vi "Sensor_Save.vi"(0 "ED33_output":string[][](array[string]), 1 "Sensor_output":string[][](array[string]), 2 "ED33 Active?":bool, 3 "Current Cordinates":T1 {"Schritte B" format="%#.4g"; "Schritte A" format="%#.4g"; "Schritte C" format="%#.4g"; "Schritte U" format="%#.4g"; "Z axis" format="%#.4g"; "Y axis" format="%#.4g"; "X axis" format="%#.4g"}, 4 "Sensor Box":string(combo), 5 "Cont/MM":string(combo)="Continuous", 6 "Sensors Active?":bool, 7 "Min_move":dbl) -> ()   [LabVIEW 2013]
uses:
  <vilib>/express/express shared/transition.llb/Dynamic To Waveform Array.vi
  <vilib>/express/express signal manip/GetorSetDDTAttributes/Set DDT Attributes/SetT0.vi
  <vilib>/express/express shared/transition.llb/Waveform Array To Dynamic.vi
  <vilib>/express/express signal manip/GetorSetDDTAttributes/Set DDT Attributes/Set DDT Properties.xnode
panel:
  out "error out 2":errorcluster caption="error out"
  in  "error in (no error)":errorcluster
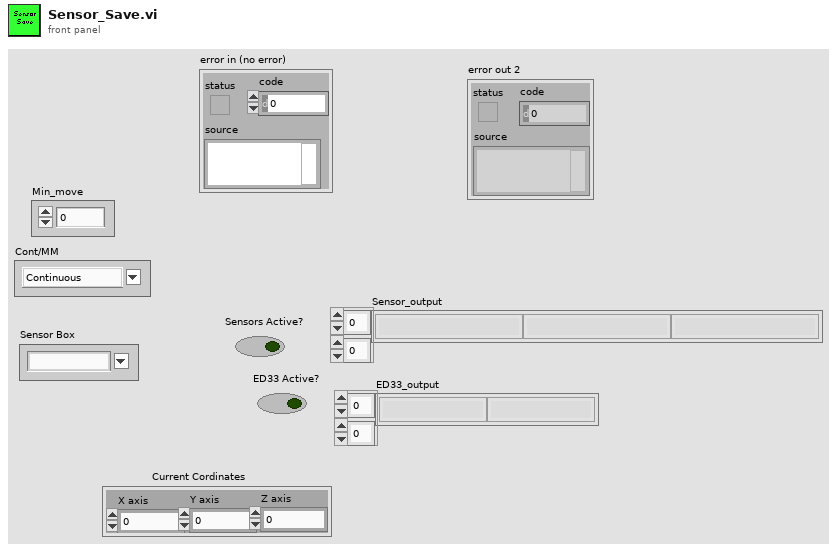
[diagram p1: front panel]
types:
  T1 = cluster{"X axis":sgl, "Y axis":sgl, "Z axis":sgl, "Schritte U":sgl, "Schritte C":sgl, "Schritte A":sgl, "Schritte B":sgl}
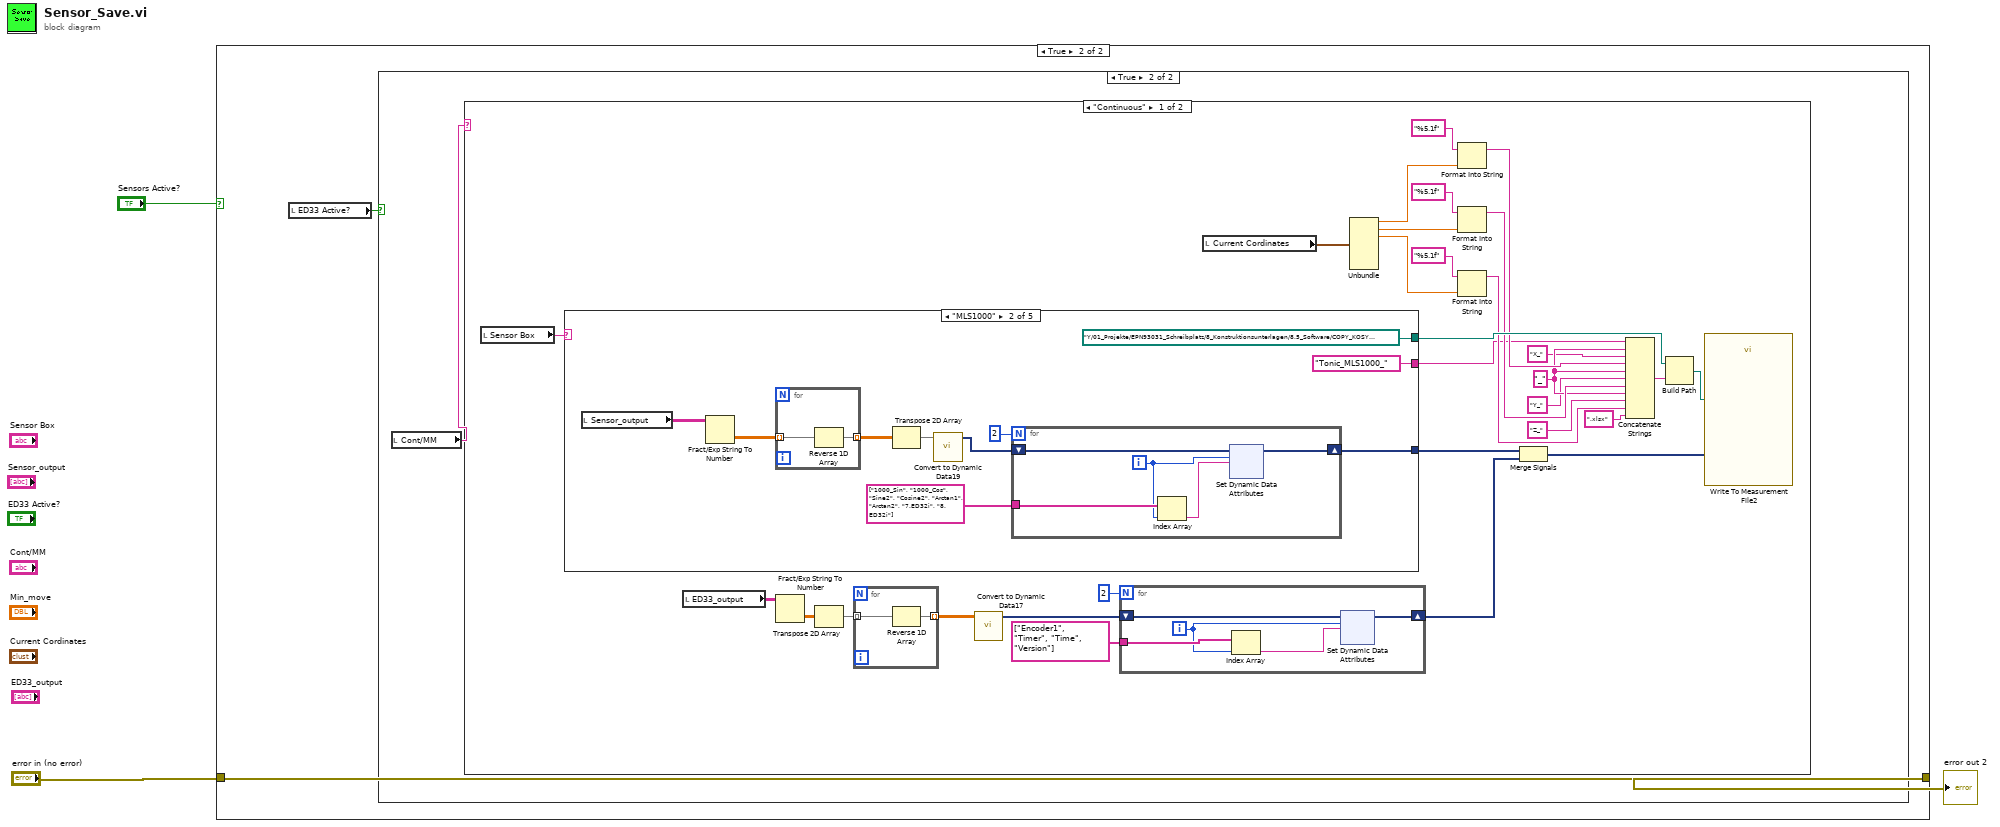
[diagram p0: block diagram]
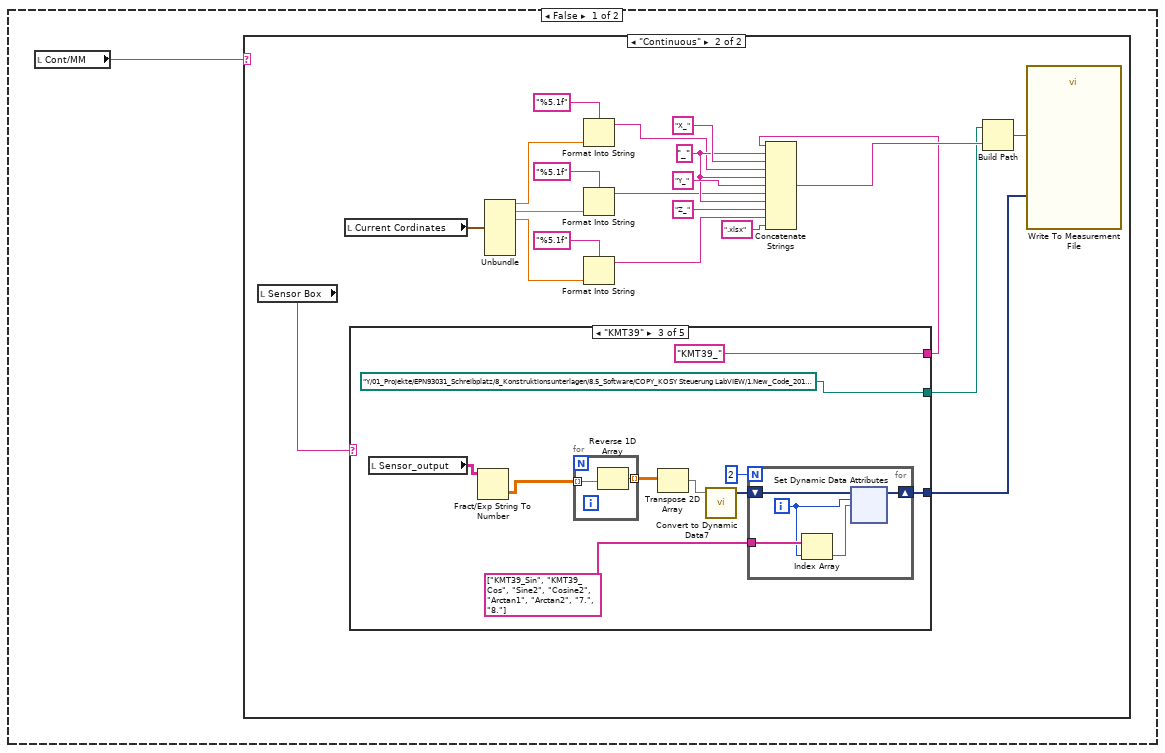
[diagram p3: hidden frame]
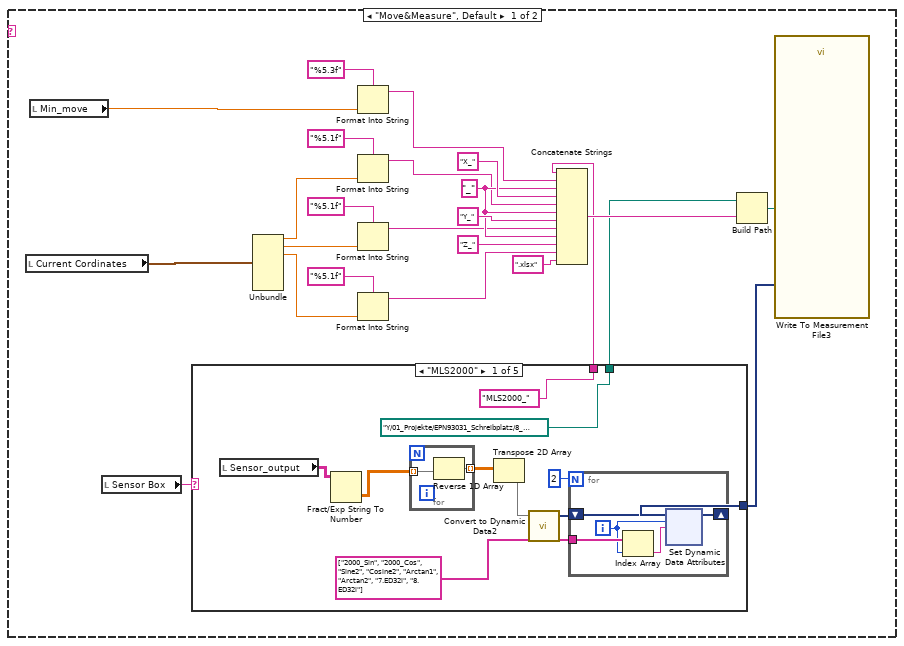
[diagram p4: hidden frame]
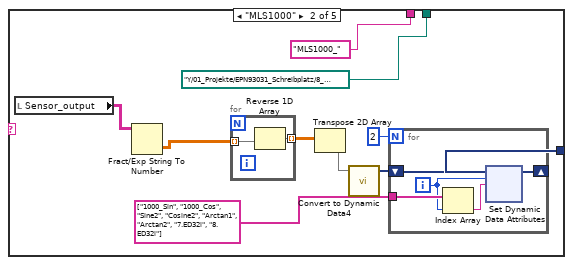
[diagram p5: hidden frame]
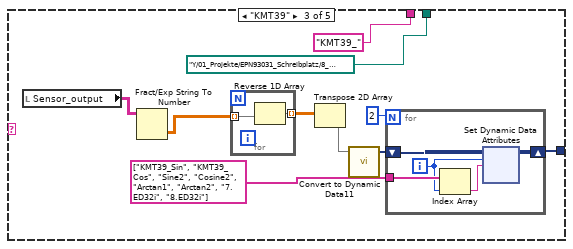
[diagram p6: hidden frame]
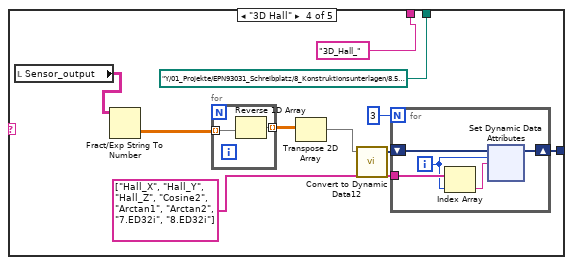
[diagram p7: hidden frame]
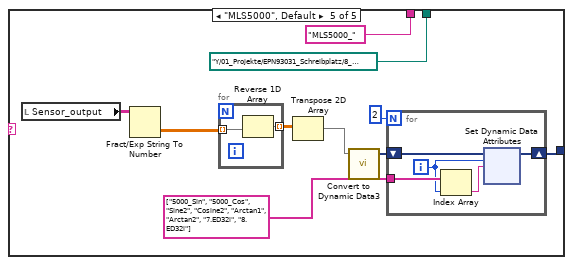
[diagram p8: hidden frame]
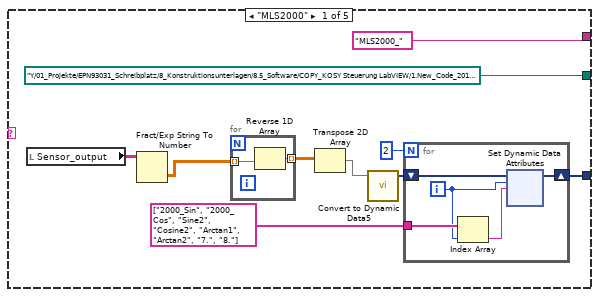
[diagram p9: hidden frame]
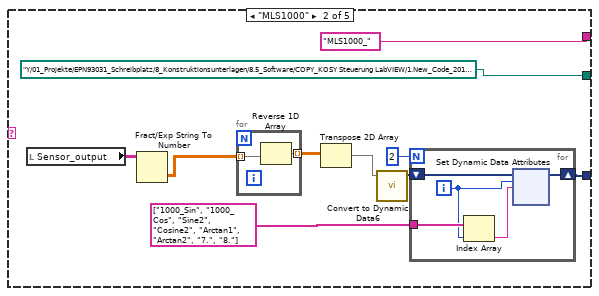
[diagram p10: hidden frame]
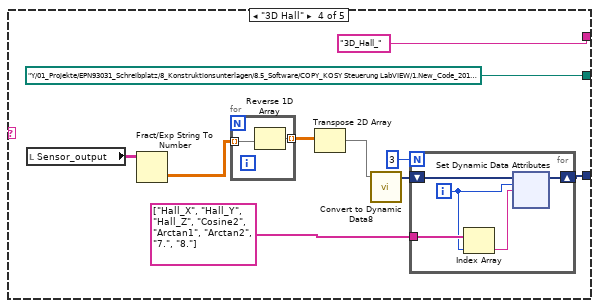
[diagram p11: hidden frame]
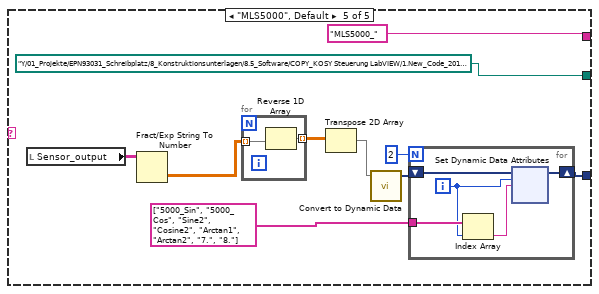
[diagram p12: hidden frame]
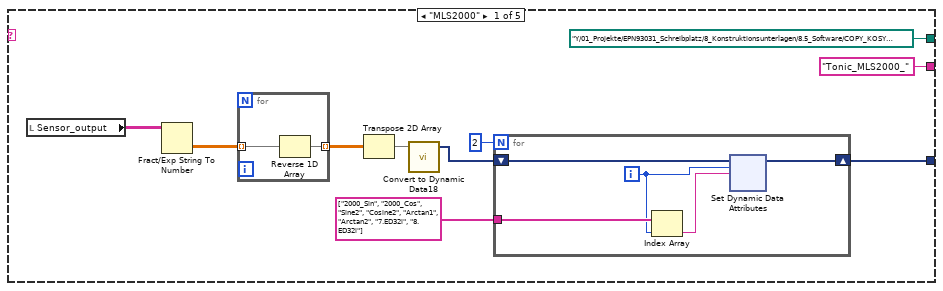
[diagram p13: hidden frame]
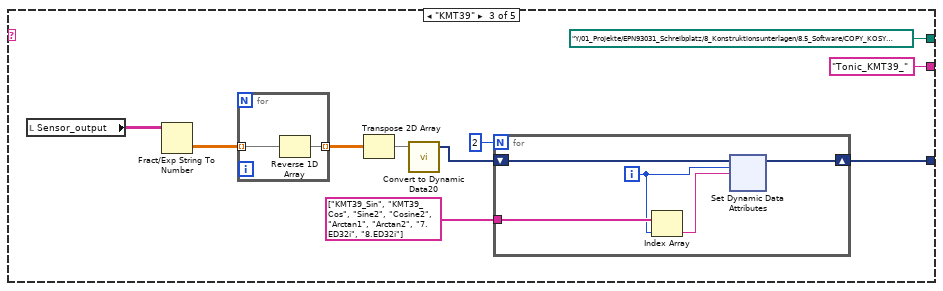
[diagram p14: hidden frame]
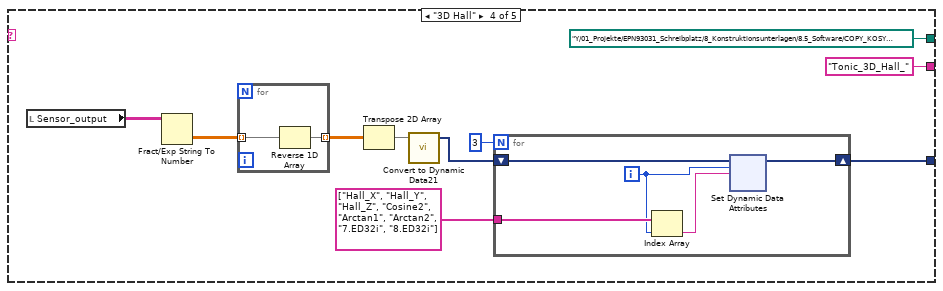
[diagram p15: hidden frame]
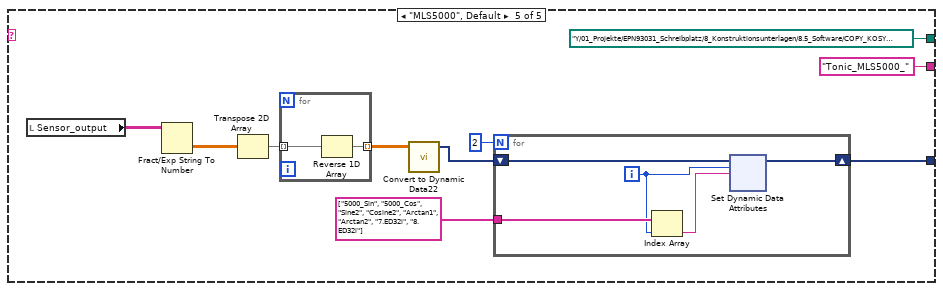
[diagram p16: hidden frame]
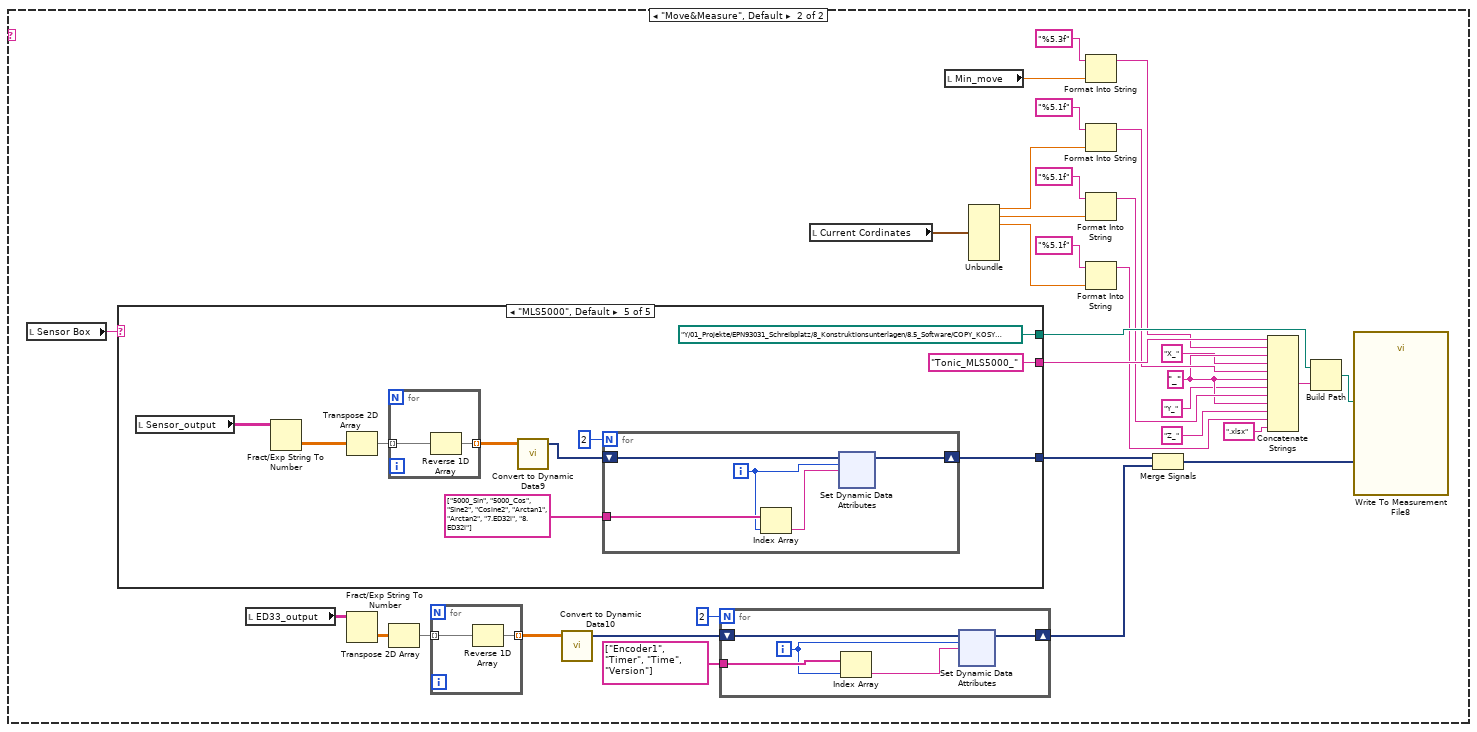
[diagram p17: hidden frame]
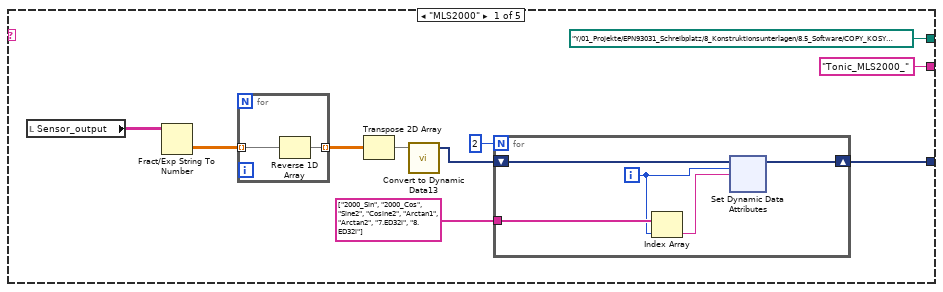
[diagram p18: hidden frame]
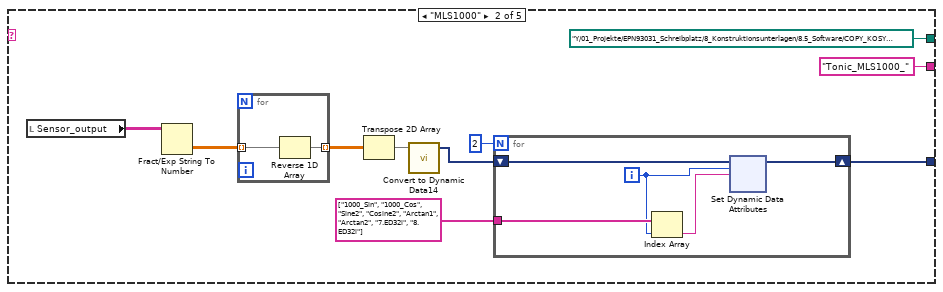
[diagram p19: hidden frame]
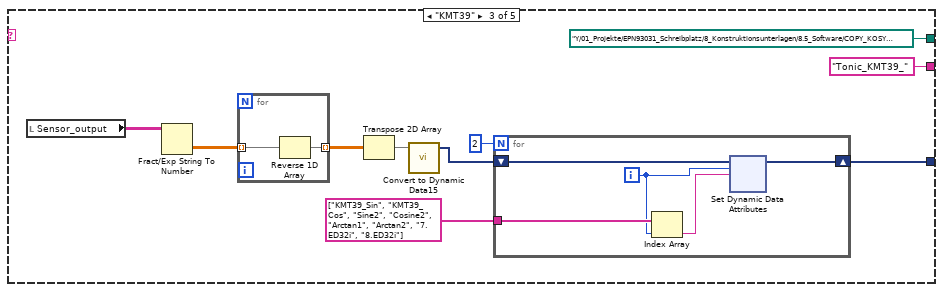
[diagram p20: hidden frame]
diagram:
  n1 = case shown="True" "Sensors Active?" {
    tunnel: "error in (no error)" -> [w4 w6]
    tunnel: [w4 w6] -> w3
    frame False {
    }
    frame True {
      n2 = local read "ED33 Active?"() -> (w5:bool)
      n3 = case shown="True" w5 {
        frame False {
          n4 = local read "Cont/MM"() -> (w7:string)
          n5 = case shown="\"Continuous\"" w7 {
            frame "Move&Measure", Default {
              w23 = "_" ("name or relative path")
              n6 = local read "Current Cordinates"() -> (w28:T1)
              n7 = local read "Min_move"() -> (w21:dbl)
              n8 = local read "Sensor Box"() -> (w10:string)
              n9 = case shown="\"MLS2000\"" w10 {
                tunnel: [w37 w67 w96 w128 w160] -> w31
                tunnel: [path "Y:/01_Projekte/EPN93031_Schreibplatz/8_Konstruktionsunterlagen/8.5_Software/COPY_KOSY Steuerung LabVIEW/1.New_Code_2014_2015/Sample_Data_ED33_32i/move&measure/MLS2000" ("base path") path "Y:/01_Projekte/EPN93031_Schreibplatz/8_Konstruktionsunterlagen/8.5_Software/COPY_KOSY Steuerung LabVIEW/1.New_Code_2014_2015/Sample_Data_ED33_32i/move&measure/MLS1000" ("base path") path "Y:/01_Projekte/EPN93031_Schreibplatz/8_Konstruktionsunterlagen/8.5_Software/COPY_KOSY Steuerung LabVIEW/1.New_Code_2014_2015/Sample_Data_ED33_32i/move&measure/KMT39" ("base path") path "Y:/01_Projekte/EPN93031_Schreibplatz/8_Konstruktionsunterlagen/8.5_Software/COPY_KOSY Steuerung LabVIEW/1.New_Code_2014_2015/Sample_Data_ED33_32i/move&measure/3D_Hall" ("base path") path "Y:/01_Projekte/EPN93031_Schreibplatz/8_Konstruktionsunterlagen/8.5_Software/COPY_KOSY Steuerung LabVIEW/1.New_Code_2014_2015/Sample_Data_ED33_32i/move&measure/MLS5000" ("base path")] -> w9
                tunnel: ["MLS2000_" ("name or relative path") "MLS1000_" ("name or relative path") "KMT39_" ("name or relative path") "3D_Hall_" ("name or relative path") "MLS5000_" ("name or relative path")] -> w8
                frame "MLS2000" {
                  n10 = local read "Sensor_output"() -> (w36:string[][])
                  n11 = Fract/Exp String To Number(string=w36) -> (number=w32:dbl[][])  [unwired: 3 in, 1 out]
                  n12 = for {
                    tunnel: w32 -> [w43] mode=indexing
                    tunnel: [w42] -> w34 mode=indexing
                    n13 = Reverse 1D Array(array=w43) -> (reversed array=w42:dbl[])
                  }
                  n14 = Transpose 2D Array(2D array=w34) -> (transposed array=w33:dbl[][])
                  n15 = call "Convert to Dynamic Data2"("2D Array"=w33) -> ("Dynamic Data Type"=w39:dynamicdata)  [unwired: 3 in]
                  n16 = for {
                    N: 2 -> [_]
                    tunnel: string[] ["2000_Sin", "2000_Cos", "Sine2", "Cosine2", "Arctan1", "Arctan2", "7.ED32i", "8.ED32i"] -> [w48]
                    shift-right: [w45] -> w37
                    shift-left: w39 -> [w44]
                    i -> [w46]
                    n17 = Index Array(array=w48, index=w46) -> (element=w47:string)
                    n18 = xnode ("Set Dynamic Data Attributes")("Signals In"=w44, "Signal Index"=w46, "Signal Name"=w47) -> ("Signals Out"=w45:dynamicdata)  [unwired: 1 in, 1 out]
                  }
                }
                frame "MLS1000" {
                  n19 = local read "Sensor_output"() -> (w68:string[][])
                  n20 = Fract/Exp String To Number(string=w68) -> (number=w62:dbl[][])  [unwired: 3 in, 1 out]
                  n21 = for {
                    tunnel: w62 -> [w73] mode=indexing
                    tunnel: [w72] -> w64 mode=indexing
                    n22 = Reverse 1D Array(array=w73) -> (reversed array=w72:dbl[])
                  }
                  n23 = Transpose 2D Array(2D array=w64) -> (transposed array=w63:dbl[][])
                  n24 = call "Convert to Dynamic Data4"("2D Array"=w63) -> ("Dynamic Data Type"=w69:dynamicdata)  [unwired: 3 in]
                  n25 = for {
                    N: 2 -> [_]
                    tunnel: string[] ["1000_Sin", "1000_Cos", "Sine2", "Cosine2", "Arctan1", "Arctan2", "7.ED32i", "8.ED32i"] -> [w78]
                    shift-right: [w75] -> w67
                    shift-left: w69 -> [w74]
                    i -> [w76]
                    n26 = Index Array(array=w78, index=w76) -> (element=w77:string)
                    n27 = xnode ("Set Dynamic Data Attributes")("Signals In"=w74, "Signal Index"=w76, "Signal Name"=w77) -> ("Signals Out"=w75:dynamicdata)  [unwired: 1 in, 1 out]
                  }
                }
                frame "KMT39" {
                  n28 = local read "Sensor_output"() -> (w98:string[][])
                  n29 = Fract/Exp String To Number(string=w98) -> (number=w92:dbl[][])  [unwired: 3 in, 1 out]
                  n30 = for {
                    tunnel: w92 -> [w103] mode=indexing
                    tunnel: [w102] -> w94 mode=indexing
                    n31 = Reverse 1D Array(array=w103) -> (reversed array=w102:dbl[])
                  }
                  n32 = Transpose 2D Array(2D array=w94) -> (transposed array=w93:dbl[][])
                  n33 = call "Convert to Dynamic Data11"("2D Array"=w93) -> ("Dynamic Data Type"=w99:dynamicdata)  [unwired: 3 in]
                  n34 = for {
                    N: 2 -> [_]
                    tunnel: string[] ["KMT39_Sin", "KMT39_Cos", "Sine2", "Cosine2", "Arctan1", "Arctan2", "7.ED32i", "8.ED32i"] -> [w108]
                    shift-right: [w105] -> w96
                    shift-left: w99 -> [w104]
                    i -> [w106]
                    n35 = Index Array(array=w108, index=w106) -> (element=w107:string)
                    n36 = xnode ("Set Dynamic Data Attributes")("Signals In"=w104, "Signal Index"=w106, "Signal Name"=w107) -> ("Signals Out"=w105:dynamicdata)  [unwired: 1 in, 1 out]
                  }
                }
                frame "3D Hall" {
                  n37 = local read "Sensor_output"() -> (w126:string[][])
                  n38 = Fract/Exp String To Number(string=w126) -> (number=w122:dbl[][])  [unwired: 3 in, 1 out]
                  n39 = for {
                    tunnel: w122 -> [w133] mode=indexing
                    tunnel: [w132] -> w124 mode=indexing
                    n40 = Reverse 1D Array(array=w133) -> (reversed array=w132:dbl[])
                  }
                  n41 = Transpose 2D Array(2D array=w124) -> (transposed array=w123:dbl[][])
                  n42 = call "Convert to Dynamic Data12"("2D Array"=w123) -> ("Dynamic Data Type"=w129:dynamicdata)  [unwired: 3 in]
                  n43 = for {
                    N: 3 -> [_]
                    tunnel: string[] ["Hall_X", "Hall_Y", "Hall_Z", "Cosine2", "Arctan1", "Arctan2", "7.ED32i", "8.ED32i"] -> [w138]
                    shift-right: [w135] -> w128
                    shift-left: w129 -> [w134]
                    i -> [w136]
                    n44 = Index Array(array=w138, index=w136) -> (element=w137:string)
                    n45 = xnode ("Set Dynamic Data Attributes")("Signals In"=w134, "Signal Index"=w136, "Signal Name"=w137) -> ("Signals Out"=w135:dynamicdata)  [unwired: 1 in, 1 out]
                  }
                }
                frame "MLS5000", Default {
                  n46 = local read "Sensor_output"() -> (w157:string[][])
                  n47 = Fract/Exp String To Number(string=w157) -> (number=w152:dbl[][])  [unwired: 3 in, 1 out]
                  n48 = for {
                    tunnel: w152 -> [w163] mode=indexing
                    tunnel: [w162] -> w154 mode=indexing
                    n49 = Reverse 1D Array(array=w163) -> (reversed array=w162:dbl[])
                  }
                  n50 = Transpose 2D Array(2D array=w154) -> (transposed array=w153:dbl[][])
                  n51 = call "Convert to Dynamic Data3"("2D Array"=w153) -> ("Dynamic Data Type"=w161:dynamicdata)  [unwired: 3 in]
                  n52 = for {
                    N: 2 -> [_]
                    tunnel: string[] ["5000_Sin", "5000_Cos", "Sine2", "Cosine2", "Arctan1", "Arctan2", "7.ED32i", "8.ED32i"] -> [w168]
                    shift-right: [w165] -> w160
                    shift-left: w161 -> [w164]
                    i -> [w166]
                    n53 = Index Array(array=w168, index=w166) -> (element=w167:string)
                    n54 = xnode ("Set Dynamic Data Attributes")("Signals In"=w164, "Signal Index"=w166, "Signal Name"=w167) -> ("Signals Out"=w165:dynamicdata)  [unwired: 1 in, 1 out]
                  }
                }
              }
              n55 = Unbundle(w28) -> ("X axis"=w16:sgl, "Y axis"=w15:sgl, "Z axis"=w14:sgl)  [unwired: 4 out]
              n56 = Format Into String(format string="%5.3f", w21) -> (resulting string=w20:string)  [unwired: 2 in, 1 out]
              n57 = Format Into String(format string="%5.1f", w16) -> (resulting string=w13:string)  [unwired: 2 in, 1 out]
              n58 = Format Into String(format string="%5.1f", w15) -> (resulting string=w12:string)  [unwired: 2 in, 1 out]
              n59 = Format Into String(format string="%5.1f", w14) -> (resulting string=w11:string)  [unwired: 2 in, 1 out]
              n60 = Concatenate Strings(w8, w20, w23, "X_" ("name or relative path"), w13, w23, "Y_" ("name or relative path"), w12, w23, "Z_" ("name or relative path"), w11, ".xlsx" ("name or relative path")) -> (w30:string)
              n61 = Build Path(base path=w9, name or relative path=w30) -> (appended path=w29:path)
              n62 = call "Write To Measurement File3"("Signals"=w31, "Filename"=w29) -> ()  [unwired: 15 in, 3 out]
            }
            frame "Continuous" {
              w196 = "_" ("name or relative path")
              n63 = local read "Sensor Box"() -> (w184:string)
              n64 = local read "Current Cordinates"() -> (w186:T1)
              n65 = case shown="\"KMT39\"" w184 {
                tunnel: [w208 w238 w269 w298 w331] -> w202
                tunnel: [path "Y:/01_Projekte/EPN93031_Schreibplatz/8_Konstruktionsunterlagen/8.5_Software/COPY_KOSY Steuerung LabVIEW/1.New_Code_2014_2015/Sample_Data_ED33_32i/continuous/MLS2000" ("base path") path "Y:/01_Projekte/EPN93031_Schreibplatz/8_Konstruktionsunterlagen/8.5_Software/COPY_KOSY Steuerung LabVIEW/1.New_Code_2014_2015/Sample_Data_ED33_32i/continuous/MLS1000" ("base path") path "Y:/01_Projekte/EPN93031_Schreibplatz/8_Konstruktionsunterlagen/8.5_Software/COPY_KOSY Steuerung LabVIEW/1.New_Code_2014_2015/Sample_Data_ED33_32i/continuous/KMT39" ("base path") path "Y:/01_Projekte/EPN93031_Schreibplatz/8_Konstruktionsunterlagen/8.5_Software/COPY_KOSY Steuerung LabVIEW/1.New_Code_2014_2015/Sample_Data_ED33_32i/continuous/3D_Hall" ("base path") path "Y:/01_Projekte/EPN93031_Schreibplatz/8_Konstruktionsunterlagen/8.5_Software/COPY_KOSY Steuerung LabVIEW/1.New_Code_2014_2015/Sample_Data_ED33_32i/continuous/MLS5000" ("base path")] -> w183
                tunnel: ["MLS2000_" ("name or relative path") "MLS1000_" ("name or relative path") "KMT39_" ("name or relative path") "3D_Hall_" ("name or relative path") "MLS5000_" ("name or relative path")] -> w182
                frame "MLS2000" {
                  n66 = local read "Sensor_output"() -> (w209:string[][])
                  n67 = Fract/Exp String To Number(string=w209) -> (number=w203:dbl[][])  [unwired: 3 in, 1 out]
                  n68 = for {
                    tunnel: w203 -> [w214] mode=indexing
                    tunnel: [w213] -> w205 mode=indexing
                    n69 = Reverse 1D Array(array=w214) -> (reversed array=w213:dbl[])
                  }
                  n70 = Transpose 2D Array(2D array=w205) -> (transposed array=w204:dbl[][])
                  n71 = call "Convert to Dynamic Data5"("2D Array"=w204) -> ("Dynamic Data Type"=w212:dynamicdata)  [unwired: 3 in]
                  n72 = for {
                    N: 2 -> [_]
                    tunnel: string[] ["2000_Sin", "2000_Cos", "Sine2", "Cosine2", "Arctan1", "Arctan2", "7.", "8."] -> [w219]
                    shift-right: [w216] -> w208
                    shift-left: w212 -> [w215]
                    i -> [w217]
                    n73 = Index Array(array=w219, index=w217) -> (element=w218:string)
                    n74 = xnode ("Set Dynamic Data Attributes")("Signals In"=w215, "Signal Index"=w217, "Signal Name"=w218) -> ("Signals Out"=w216:dynamicdata)  [unwired: 1 in, 1 out]
                  }
                }
                frame "MLS1000" {
                  n75 = local read "Sensor_output"() -> (w239:string[][])
                  n76 = Fract/Exp String To Number(string=w239) -> (number=w233:dbl[][])  [unwired: 3 in, 1 out]
                  n77 = for {
                    tunnel: w233 -> [w244] mode=indexing
                    tunnel: [w243] -> w235 mode=indexing
                    n78 = Reverse 1D Array(array=w244) -> (reversed array=w243:dbl[])
                  }
                  n79 = Transpose 2D Array(2D array=w235) -> (transposed array=w234:dbl[][])
                  n80 = call "Convert to Dynamic Data6"("2D Array"=w234) -> ("Dynamic Data Type"=w242:dynamicdata)  [unwired: 3 in]
                  n81 = for {
                    N: 2 -> [_]
                    tunnel: string[] ["1000_Sin", "1000_Cos", "Sine2", "Cosine2", "Arctan1", "Arctan2", "7.", "8."] -> [w249]
                    shift-right: [w246] -> w238
                    shift-left: w242 -> [w245]
                    i -> [w247]
                    n82 = Index Array(array=w249, index=w247) -> (element=w248:string)
                    n83 = xnode ("Set Dynamic Data Attributes")("Signals In"=w245, "Signal Index"=w247, "Signal Name"=w248) -> ("Signals Out"=w246:dynamicdata)  [unwired: 1 in, 1 out]
                  }
                }
                frame "KMT39" {
                  n84 = local read "Sensor_output"() -> (w266:string[][])
                  n85 = Fract/Exp String To Number(string=w266) -> (number=w263:dbl[][])  [unwired: 3 in, 1 out]
                  n86 = for {
                    tunnel: w263 -> [w274] mode=indexing
                    tunnel: [w273] -> w265 mode=indexing
                    n87 = Reverse 1D Array(array=w274) -> (reversed array=w273:dbl[])
                  }
                  n88 = Transpose 2D Array(2D array=w265) -> (transposed array=w264:dbl[][])
                  n89 = call "Convert to Dynamic Data7"("2D Array"=w264) -> ("Dynamic Data Type"=w270:dynamicdata)  [unwired: 3 in]
                  n90 = for {
                    N: 2 -> [_]
                    tunnel: string[] ["KMT39_Sin", "KMT39_Cos", "Sine2", "Cosine2", "Arctan1", "Arctan2", "7.", "8."] -> [w279]
                    shift-right: [w276] -> w269
                    shift-left: w270 -> [w275]
                    i -> [w277]
                    n91 = Index Array(array=w279, index=w277) -> (element=w278:string)
                    n92 = xnode ("Set Dynamic Data Attributes")("Signals In"=w275, "Signal Index"=w277, "Signal Name"=w278) -> ("Signals Out"=w276:dynamicdata)  [unwired: 1 in, 1 out]
                  }
                }
                frame "3D Hall" {
                  n93 = local read "Sensor_output"() -> (w299:string[][])
                  n94 = Fract/Exp String To Number(string=w299) -> (number=w293:dbl[][])  [unwired: 3 in, 1 out]
                  n95 = for {
                    tunnel: w293 -> [w304] mode=indexing
                    tunnel: [w303] -> w295 mode=indexing
                    n96 = Reverse 1D Array(array=w304) -> (reversed array=w303:dbl[])
                  }
                  n97 = Transpose 2D Array(2D array=w295) -> (transposed array=w294:dbl[][])
                  n98 = call "Convert to Dynamic Data8"("2D Array"=w294) -> ("Dynamic Data Type"=w302:dynamicdata)  [unwired: 3 in]
                  n99 = for {
                    N: 3 -> [_]
                    tunnel: string[] ["Hall_X", "Hall_Y", "Hall_Z", "Cosine2", "Arctan1", "Arctan2", "7.", "8."] -> [w309]
                    shift-right: [w306] -> w298
                    shift-left: w302 -> [w305]
                    i -> [w307]
                    n100 = Index Array(array=w309, index=w307) -> (element=w308:string)
                    n101 = xnode ("Set Dynamic Data Attributes")("Signals In"=w305, "Signal Index"=w307, "Signal Name"=w308) -> ("Signals Out"=w306:dynamicdata)  [unwired: 1 in, 1 out]
                  }
                }
                frame "MLS5000", Default {
                  n102 = local read "Sensor_output"() -> (w328:string[][])
                  n103 = Fract/Exp String To Number(string=w328) -> (number=w323:dbl[][])  [unwired: 3 in, 1 out]
                  n104 = for {
                    tunnel: w323 -> [w334] mode=indexing
                    tunnel: [w333] -> w325 mode=indexing
                    n105 = Reverse 1D Array(array=w334) -> (reversed array=w333:dbl[])
                  }
                  n106 = Transpose 2D Array(2D array=w325) -> (transposed array=w324:dbl[][])
                  n107 = call "Convert to Dynamic Data"("2D Array"=w324) -> ("Dynamic Data Type"=w332:dynamicdata)  [unwired: 3 in]
                  n108 = for {
                    N: 2 -> [_]
                    tunnel: string[] ["5000_Sin", "5000_Cos", "Sine2", "Cosine2", "Arctan1", "Arctan2", "7.", "8."] -> [w339]
                    shift-right: [w336] -> w331
                    shift-left: w332 -> [w335]
                    i -> [w337]
                    n109 = Index Array(array=w339, index=w337) -> (element=w338:string)
                    n110 = xnode ("Set Dynamic Data Attributes")("Signals In"=w335, "Signal Index"=w337, "Signal Name"=w338) -> ("Signals Out"=w336:dynamicdata)  [unwired: 1 in, 1 out]
                  }
                }
              }
              n111 = Unbundle(w186) -> ("X axis"=w192:sgl, "Y axis"=w191:sgl, "Z axis"=w190:sgl)  [unwired: 4 out]
              n112 = Format Into String(format string="%5.1f", w192) -> (resulting string=w189:string)  [unwired: 2 in, 1 out]
              n113 = Format Into String(format string="%5.1f", w191) -> (resulting string=w188:string)  [unwired: 2 in, 1 out]
              n114 = Format Into String(format string="%5.1f", w190) -> (resulting string=w187:string)  [unwired: 2 in, 1 out]
              n115 = Concatenate Strings(w182, w196, "X_" ("name or relative path"), w189, w196, "Y_" ("name or relative path"), w188, w196, "Z_" ("name or relative path"), w187, ".xlsx" ("name or relative path")) -> (w201:string)
              n116 = Build Path(base path=w183, name or relative path=w201) -> (appended path=w185:path)
              n117 = call "Write To Measurement File"("Signals"=w202, "Filename"=w185) -> ()  [unwired: 15 in, 3 out]
            }
          }
        }
        frame True {
          n118 = local read "Cont/MM"() -> (w353:string)
          n119 = case shown="\"Continuous\"" w353 {
            frame "Continuous" {
              w371 = "_" ("name or relative path")
              n120 = local read "Sensor Box"() -> (w365:string)
              n121 = case shown="\"MLS1000\"" w365 {
                tunnel: [w392 w421 w451 w481 w515] -> w359
                tunnel: [path "Y:/01_Projekte/EPN93031_Schreibplatz/8_Konstruktionsunterlagen/8.5_Software/COPY_KOSY Steuerung LabVIEW/1.New_Code_2014_2015/Sample_Data_ED33_32i/continuous/With_Ref/MLS2000" ("base path") path "Y:/01_Projekte/EPN93031_Schreibplatz/8_Konstruktionsunterlagen/8.5_Software/COPY_KOSY Steuerung LabVIEW/1.New_Code_2014_2015/Sample_Data_ED33_32i/continuous/With_Ref/MLS1000" ("base path") path "Y:/01_Projekte/EPN93031_Schreibplatz/8_Konstruktionsunterlagen/8.5_Software/COPY_KOSY Steuerung LabVIEW/1.New_Code_2014_2015/Sample_Data_ED33_32i/continuous/With_Ref/KMT39" ("base path") path "Y:/01_Projekte/EPN93031_Schreibplatz/8_Konstruktionsunterlagen/8.5_Software/COPY_KOSY Steuerung LabVIEW/1.New_Code_2014_2015/Sample_Data_ED33_32i/continuous/With_Ref/3D_Hall" ("base path") path "Y:/01_Projekte/EPN93031_Schreibplatz/8_Konstruktionsunterlagen/8.5_Software/COPY_KOSY Steuerung LabVIEW/1.New_Code_2014_2015/Sample_Data_ED33_32i/continuous/With_Ref/MLS5000" ("base path")] -> w382
                tunnel: ["Tonic_MLS2000_" ("name or relative path") "Tonic_MLS1000_" ("name or relative path") "Tonic_KMT39_" ("name or relative path") "Tonic_3D_Hall_" ("name or relative path") "Tonic_MLS5000_" ("name or relative path")] -> w354
                frame "MLS2000" {
                  n122 = local read "Sensor_output"() -> (w391:string[][])
                  n123 = Fract/Exp String To Number(string=w391) -> (number=w386:dbl[][])  [unwired: 3 in, 1 out]
                  n124 = for {
                    tunnel: w386 -> [w397] mode=indexing
                    tunnel: [w396] -> w388 mode=indexing
                    n125 = Reverse 1D Array(array=w397) -> (reversed array=w396:dbl[])
                  }
                  n126 = Transpose 2D Array(2D array=w388) -> (transposed array=w387:dbl[][])
                  n127 = call "Convert to Dynamic Data18"("2D Array"=w387) -> ("Dynamic Data Type"=w394:dynamicdata)  [unwired: 3 in]
                  n128 = for {
                    N: 2 -> [_]
                    tunnel: string[] ["2000_Sin", "2000_Cos", "Sine2", "Cosine2", "Arctan1", "Arctan2", "7.ED32i", "8.ED32i"] -> [w402]
                    shift-right: [w399] -> w392
                    shift-left: w394 -> [w398]
                    i -> [w400]
                    n129 = Index Array(array=w402, index=w400) -> (element=w401:string)
                    n130 = xnode ("Set Dynamic Data Attributes")("Signals In"=w398, "Signal Index"=w400, "Signal Name"=w401) -> ("Signals Out"=w399:dynamicdata)  [unwired: 1 in, 1 out]
                  }
                }
                frame "MLS1000" {
                  n131 = local read "Sensor_output"() -> (w422:string[][])
                  n132 = Fract/Exp String To Number(string=w422) -> (number=w416:dbl[][])  [unwired: 3 in, 1 out]
                  n133 = for {
                    tunnel: w416 -> [w427] mode=indexing
                    tunnel: [w426] -> w418 mode=indexing
                    n134 = Reverse 1D Array(array=w427) -> (reversed array=w426:dbl[])
                  }
                  n135 = Transpose 2D Array(2D array=w418) -> (transposed array=w417:dbl[][])
                  n136 = call "Convert to Dynamic Data19"("2D Array"=w417) -> ("Dynamic Data Type"=w424:dynamicdata)  [unwired: 3 in]
                  n137 = for {
                    N: 2 -> [_]
                    tunnel: string[] ["1000_Sin", "1000_Cos", "Sine2", "Cosine2", "Arctan1", "Arctan2", "7.ED32i", "8.ED32i"] -> [w432]
                    shift-right: [w429] -> w421
                    shift-left: w424 -> [w428]
                    i -> [w430]
                    n138 = Index Array(array=w432, index=w430) -> (element=w431:string)
                    n139 = xnode ("Set Dynamic Data Attributes")("Signals In"=w428, "Signal Index"=w430, "Signal Name"=w431) -> ("Signals Out"=w429:dynamicdata)  [unwired: 1 in, 1 out]
                  }
                }
                frame "KMT39" {
                  n140 = local read "Sensor_output"() -> (w452:string[][])
                  n141 = Fract/Exp String To Number(string=w452) -> (number=w446:dbl[][])  [unwired: 3 in, 1 out]
                  n142 = for {
                    tunnel: w446 -> [w457] mode=indexing
                    tunnel: [w456] -> w448 mode=indexing
                    n143 = Reverse 1D Array(array=w457) -> (reversed array=w456:dbl[])
                  }
                  n144 = Transpose 2D Array(2D array=w448) -> (transposed array=w447:dbl[][])
                  n145 = call "Convert to Dynamic Data20"("2D Array"=w447) -> ("Dynamic Data Type"=w454:dynamicdata)  [unwired: 3 in]
                  n146 = for {
                    N: 2 -> [_]
                    tunnel: string[] ["KMT39_Sin", "KMT39_Cos", "Sine2", "Cosine2", "Arctan1", "Arctan2", "7.ED32i", "8.ED32i"] -> [w462]
                    shift-right: [w459] -> w451
                    shift-left: w454 -> [w458]
                    i -> [w460]
                    n147 = Index Array(array=w462, index=w460) -> (element=w461:string)
                    n148 = xnode ("Set Dynamic Data Attributes")("Signals In"=w458, "Signal Index"=w460, "Signal Name"=w461) -> ("Signals Out"=w459:dynamicdata)  [unwired: 1 in, 1 out]
                  }
                }
                frame "3D Hall" {
                  n149 = local read "Sensor_output"() -> (w482:string[][])
                  n150 = Fract/Exp String To Number(string=w482) -> (number=w476:dbl[][])  [unwired: 3 in, 1 out]
                  n151 = for {
                    tunnel: w476 -> [w487] mode=indexing
                    tunnel: [w486] -> w478 mode=indexing
                    n152 = Reverse 1D Array(array=w487) -> (reversed array=w486:dbl[])
                  }
                  n153 = Transpose 2D Array(2D array=w478) -> (transposed array=w477:dbl[][])
                  n154 = call "Convert to Dynamic Data21"("2D Array"=w477) -> ("Dynamic Data Type"=w484:dynamicdata)  [unwired: 3 in]
                  n155 = for {
                    N: 3 -> [_]
                    tunnel: string[] ["Hall_X", "Hall_Y", "Hall_Z", "Cosine2", "Arctan1", "Arctan2", "7.ED32i", "8.ED32i"] -> [w492]
                    shift-right: [w489] -> w481
                    shift-left: w484 -> [w488]
                    i -> [w490]
                    n156 = Index Array(array=w492, index=w490) -> (element=w491:string)
                    n157 = xnode ("Set Dynamic Data Attributes")("Signals In"=w488, "Signal Index"=w490, "Signal Name"=w491) -> ("Signals Out"=w489:dynamicdata)  [unwired: 1 in, 1 out]
                  }
                }
                frame "MLS5000", Default {
                  n158 = local read "Sensor_output"() -> (w514:string[][])
                  n159 = Fract/Exp String To Number(string=w514) -> (number=w507:dbl[][])  [unwired: 3 in, 1 out]
                  n160 = Transpose 2D Array(2D array=w507) -> (transposed array=w506:dbl[][])
                  n161 = for {
                    tunnel: w506 -> [w517] mode=indexing
                    tunnel: [w516] -> w508 mode=indexing
                    n162 = Reverse 1D Array(array=w517) -> (reversed array=w516:dbl[])
                  }
                  n163 = call "Convert to Dynamic Data22"("2D Array"=w508) -> ("Dynamic Data Type"=w512:dynamicdata)  [unwired: 3 in]
                  n164 = for {
                    N: 2 -> [_]
                    tunnel: string[] ["5000_Sin", "5000_Cos", "Sine2", "Cosine2", "Arctan1", "Arctan2", "7.ED32i", "8.ED32i"] -> [w522]
                    shift-right: [w519] -> w515
                    shift-left: w512 -> [w518]
                    i -> [w520]
                    n165 = Index Array(array=w522, index=w520) -> (element=w521:string)
                    n166 = xnode ("Set Dynamic Data Attributes")("Signals In"=w518, "Signal Index"=w520, "Signal Name"=w521) -> ("Signals Out"=w519:dynamicdata)  [unwired: 1 in, 1 out]
                  }
                }
              }
              n167 = local read "ED33_output"() -> (w361:string[][])
              n168 = Fract/Exp String To Number(string=w361) -> (number=w356:dbl[][])  [unwired: 3 in, 1 out]
              n169 = Transpose 2D Array(2D array=w356) -> (transposed array=w355:dbl[][])
              n170 = for {
                tunnel: w355 -> [w385] mode=indexing
                tunnel: [w384] -> w357 mode=indexing
                n171 = Reverse 1D Array(array=w385) -> (reversed array=w384:dbl[])
              }
              n172 = call "Convert to Dynamic Data17"("2D Array"=w357) -> ("Dynamic Data Type"=w362:dynamicdata)  [unwired: 3 in]
              n173 = for {
                N: 2 -> [_]
                tunnel: string[] ["Encoder1", "Timer", "Time", "Version"] -> [w540]
                shift-right: [w537] -> w360
                shift-left: w362 -> [w536]
                i -> [w538]
                n174 = Index Array(array=w540, index=w538) -> (element=w539:string)
                n175 = xnode ("Set Dynamic Data Attributes")("Signals In"=w536, "Signal Index"=w538, "Signal Name"=w539) -> ("Signals Out"=w537:dynamicdata)  [unwired: 1 in, 1 out]
              }
              n176 = local read "Current Cordinates"() -> (w381:T1)
              n177 = Unbundle(w381) -> ("X axis"=w375:sgl, "Y axis"=w376:sgl, "Z axis"=w377:sgl)  [unwired: 4 out]
              n178 = Format Into String(format string="%5.1f", w375) -> (resulting string=w378:string)  [unwired: 2 in, 1 out]
              n179 = Format Into String(format string="%5.1f", w376) -> (resulting string=w379:string)  [unwired: 2 in, 1 out]
              n180 = Format Into String(format string="%5.1f", w377) -> (resulting string=w380:string)  [unwired: 2 in, 1 out]
              n181 = Merge Signals(w359, w360) -> (w358:dynamicdata)
              n182 = Concatenate Strings(w354, w371, "X_" ("name or relative path"), w378, w371, "Y_" ("name or relative path"), w379, w371, "Z_" ("name or relative path"), w380, ".xlsx" ("name or relative path")) -> (w366:string)
              n183 = Build Path(base path=w382, name or relative path=w366) -> (appended path=w383:path)
              n184 = call "Write To Measurement File2"("Signals"=w358, "Filename"=w383) -> ()  [unwired: 15 in, 3 out]
            }
            frame "Move&Measure", Default {
              w570 = "_" ("name or relative path")
              n185 = local read "Sensor Box"() -> (w564:string)
              n186 = case shown="\"MLS5000\", Default" w564 {
                tunnel: [w595 w624 w654 w684 w718] -> w558
                tunnel: [path "Y:/01_Projekte/EPN93031_Schreibplatz/8_Konstruktionsunterlagen/8.5_Software/COPY_KOSY Steuerung LabVIEW/1.New_Code_2014_2015/Sample_Data_ED33_32i/move&measure/With_Ref/MLS2000" ("base path") path "Y:/01_Projekte/EPN93031_Schreibplatz/8_Konstruktionsunterlagen/8.5_Software/COPY_KOSY Steuerung LabVIEW/1.New_Code_2014_2015/Sample_Data_ED33_32i/move&measure/With_Ref/MLS1000" ("base path") path "Y:/01_Projekte/EPN93031_Schreibplatz/8_Konstruktionsunterlagen/8.5_Software/COPY_KOSY Steuerung LabVIEW/1.New_Code_2014_2015/Sample_Data_ED33_32i/move&measure/With_Ref/KMT39" ("base path") path "Y:/01_Projekte/EPN93031_Schreibplatz/8_Konstruktionsunterlagen/8.5_Software/COPY_KOSY Steuerung LabVIEW/1.New_Code_2014_2015/Sample_Data_ED33_32i/move&measure/With_Ref/3D_Hall" ("base path") path "Y:/01_Projekte/EPN93031_Schreibplatz/8_Konstruktionsunterlagen/8.5_Software/COPY_KOSY Steuerung LabVIEW/1.New_Code_2014_2015/Sample_Data_ED33_32i/move&measure/With_Ref/MLS5000" ("base path")] -> w584
                tunnel: ["Tonic_MLS2000_" ("name or relative path") "Tonic_MLS1000_" ("name or relative path") "Tonic_KMT39_" ("name or relative path") "Tonic_3D_Hall_" ("name or relative path") "Tonic_MLS5000_" ("name or relative path")] -> w585
                frame "MLS2000" {
                  n187 = local read "Sensor_output"() -> (w594:string[][])
                  n188 = Fract/Exp String To Number(string=w594) -> (number=w589:dbl[][])  [unwired: 3 in, 1 out]
                  n189 = for {
                    tunnel: w589 -> [w600] mode=indexing
                    tunnel: [w599] -> w591 mode=indexing
                    n190 = Reverse 1D Array(array=w600) -> (reversed array=w599:dbl[])
                  }
                  n191 = Transpose 2D Array(2D array=w591) -> (transposed array=w590:dbl[][])
                  n192 = call "Convert to Dynamic Data13"("2D Array"=w590) -> ("Dynamic Data Type"=w597:dynamicdata)  [unwired: 3 in]
                  n193 = for {
                    N: 2 -> [_]
                    tunnel: string[] ["2000_Sin", "2000_Cos", "Sine2", "Cosine2", "Arctan1", "Arctan2", "7.ED32i", "8.ED32i"] -> [w605]
                    shift-right: [w602] -> w595
                    shift-left: w597 -> [w601]
                    i -> [w603]
                    n194 = Index Array(array=w605, index=w603) -> (element=w604:string)
                    n195 = xnode ("Set Dynamic Data Attributes")("Signals In"=w601, "Signal Index"=w603, "Signal Name"=w604) -> ("Signals Out"=w602:dynamicdata)  [unwired: 1 in, 1 out]
                  }
                }
                frame "MLS1000" {
                  n196 = local read "Sensor_output"() -> (w625:string[][])
                  n197 = Fract/Exp String To Number(string=w625) -> (number=w619:dbl[][])  [unwired: 3 in, 1 out]
                  n198 = for {
                    tunnel: w619 -> [w630] mode=indexing
                    tunnel: [w629] -> w621 mode=indexing
                    n199 = Reverse 1D Array(array=w630) -> (reversed array=w629:dbl[])
                  }
                  n200 = Transpose 2D Array(2D array=w621) -> (transposed array=w620:dbl[][])
                  n201 = call "Convert to Dynamic Data14"("2D Array"=w620) -> ("Dynamic Data Type"=w627:dynamicdata)  [unwired: 3 in]
                  n202 = for {
                    N: 2 -> [_]
                    tunnel: string[] ["1000_Sin", "1000_Cos", "Sine2", "Cosine2", "Arctan1", "Arctan2", "7.ED32i", "8.ED32i"] -> [w635]
                    shift-right: [w632] -> w624
                    shift-left: w627 -> [w631]
                    i -> [w633]
                    n203 = Index Array(array=w635, index=w633) -> (element=w634:string)
                    n204 = xnode ("Set Dynamic Data Attributes")("Signals In"=w631, "Signal Index"=w633, "Signal Name"=w634) -> ("Signals Out"=w632:dynamicdata)  [unwired: 1 in, 1 out]
                  }
                }
                frame "KMT39" {
                  n205 = local read "Sensor_output"() -> (w655:string[][])
                  n206 = Fract/Exp String To Number(string=w655) -> (number=w649:dbl[][])  [unwired: 3 in, 1 out]
                  n207 = for {
                    tunnel: w649 -> [w660] mode=indexing
                    tunnel: [w659] -> w651 mode=indexing
                    n208 = Reverse 1D Array(array=w660) -> (reversed array=w659:dbl[])
                  }
                  n209 = Transpose 2D Array(2D array=w651) -> (transposed array=w650:dbl[][])
                  n210 = call "Convert to Dynamic Data15"("2D Array"=w650) -> ("Dynamic Data Type"=w657:dynamicdata)  [unwired: 3 in]
                  n211 = for {
                    N: 2 -> [_]
                    tunnel: string[] ["KMT39_Sin", "KMT39_Cos", "Sine2", "Cosine2", "Arctan1", "Arctan2", "7.ED32i", "8.ED32i"] -> [w665]
                    shift-right: [w662] -> w654
                    shift-left: w657 -> [w661]
                    i -> [w663]
                    n212 = Index Array(array=w665, index=w663) -> (element=w664:string)
                    n213 = xnode ("Set Dynamic Data Attributes")("Signals In"=w661, "Signal Index"=w663, "Signal Name"=w664) -> ("Signals Out"=w662:dynamicdata)  [unwired: 1 in, 1 out]
                  }
                }
                frame "3D Hall" {
                  n214 = local read "Sensor_output"() -> (w685:string[][])
                  n215 = Fract/Exp String To Number(string=w685) -> (number=w679:dbl[][])  [unwired: 3 in, 1 out]
                  n216 = for {
                    tunnel: w679 -> [w690] mode=indexing
                    tunnel: [w689] -> w681 mode=indexing
                    n217 = Reverse 1D Array(array=w690) -> (reversed array=w689:dbl[])
                  }
                  n218 = Transpose 2D Array(2D array=w681) -> (transposed array=w680:dbl[][])
                  n219 = call "Convert to Dynamic Data16"("2D Array"=w680) -> ("Dynamic Data Type"=w687:dynamicdata)  [unwired: 3 in]
                  n220 = for {
                    N: 3 -> [_]
                    tunnel: string[] ["Hall_X", "Hall_Y", "Hall_Z", "Cosine2", "Arctan1", "Arctan2", "7.ED32i", "8.ED32i"] -> [w695]
                    shift-right: [w692] -> w684
                    shift-left: w687 -> [w691]
                    i -> [w693]
                    n221 = Index Array(array=w695, index=w693) -> (element=w694:string)
                    n222 = xnode ("Set Dynamic Data Attributes")("Signals In"=w691, "Signal Index"=w693, "Signal Name"=w694) -> ("Signals Out"=w692:dynamicdata)  [unwired: 1 in, 1 out]
                  }
                }
                frame "MLS5000", Default {
                  n223 = local read "Sensor_output"() -> (w717:string[][])
                  n224 = Fract/Exp String To Number(string=w717) -> (number=w710:dbl[][])  [unwired: 3 in, 1 out]
                  n225 = Transpose 2D Array(2D array=w710) -> (transposed array=w709:dbl[][])
                  n226 = for {
                    tunnel: w709 -> [w720] mode=indexing
                    tunnel: [w719] -> w711 mode=indexing
                    n227 = Reverse 1D Array(array=w720) -> (reversed array=w719:dbl[])
                  }
                  n228 = call "Convert to Dynamic Data9"("2D Array"=w711) -> ("Dynamic Data Type"=w715:dynamicdata)  [unwired: 3 in]
                  n229 = for {
                    N: 2 -> [_]
                    tunnel: string[] ["5000_Sin", "5000_Cos", "Sine2", "Cosine2", "Arctan1", "Arctan2", "7.ED32i", "8.ED32i"] -> [w725]
                    shift-right: [w722] -> w718
                    shift-left: w715 -> [w721]
                    i -> [w723]
                    n230 = Index Array(array=w725, index=w723) -> (element=w724:string)
                    n231 = xnode ("Set Dynamic Data Attributes")("Signals In"=w721, "Signal Index"=w723, "Signal Name"=w724) -> ("Signals Out"=w722:dynamicdata)  [unwired: 1 in, 1 out]
                  }
                }
              }
              n232 = local read "ED33_output"() -> (w560:string[][])
              n233 = Fract/Exp String To Number(string=w560) -> (number=w555:dbl[][])  [unwired: 3 in, 1 out]
              n234 = Transpose 2D Array(2D array=w555) -> (transposed array=w554:dbl[][])
              n235 = for {
                tunnel: w554 -> [w588] mode=indexing
                tunnel: [w587] -> w556 mode=indexing
                n236 = Reverse 1D Array(array=w588) -> (reversed array=w587:dbl[])
              }
              n237 = call "Convert to Dynamic Data10"("2D Array"=w556) -> ("Dynamic Data Type"=w561:dynamicdata)  [unwired: 3 in]
              n238 = for {
                N: 2 -> [_]
                tunnel: string[] ["Encoder1", "Timer", "Time", "Version"] -> [w743]
                shift-right: [w740] -> w559
                shift-left: w561 -> [w739]
                i -> [w741]
                n239 = Index Array(array=w743, index=w741) -> (element=w742:string)
                n240 = xnode ("Set Dynamic Data Attributes")("Signals In"=w739, "Signal Index"=w741, "Signal Name"=w742) -> ("Signals Out"=w740:dynamicdata)  [unwired: 1 in, 1 out]
              }
              n241 = local read "Current Cordinates"() -> (w582:T1)
              n242 = local read "Min_move"() -> (w583:dbl)
              n243 = Unbundle(w582) -> ("X axis"=w576:sgl, "Y axis"=w577:sgl, "Z axis"=w578:sgl)  [unwired: 4 out]
              n244 = Format Into String(format string="%5.3f", w583) -> (resulting string=w572:string)  [unwired: 2 in, 1 out]
              n245 = Format Into String(format string="%5.1f", w576) -> (resulting string=w579:string)  [unwired: 2 in, 1 out]
              n246 = Format Into String(format string="%5.1f", w577) -> (resulting string=w580:string)  [unwired: 2 in, 1 out]
              n247 = Format Into String(format string="%5.1f", w578) -> (resulting string=w581:string)  [unwired: 2 in, 1 out]
              n248 = Merge Signals(w558, w559) -> (w557:dynamicdata)
              n249 = Concatenate Strings(w585, w572, w570, "X_" ("name or relative path"), w579, w570, "Y_" ("name or relative path"), w580, w570, "Z_" ("name or relative path"), w581, ".xlsx" ("name or relative path")) -> (w565:string)
              n250 = Build Path(base path=w584, name or relative path=w565) -> (appended path=w586:path)
              n251 = call "Write To Measurement File8"("Signals"=w557, "Filename"=w586) -> ()  [unwired: 15 in, 3 out]
            }
          }
        }
      }
    }
  }
  "error out 2" <- w3
